vi "GV PreframeclockDelay_tick.vi"() -> ()   [LabVIEW 2017]
panel:
  in  "PreframeclockDelay_tick":u32
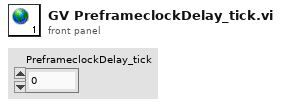
[diagram p1: front panel]
diagram:
